vi "Fit VI window to Content__ogtk.vi"(4 "error in (no error)":errorcluster, 6 "border spacing (2 px)":i32=2, 7 "VI Ref (calling VI)":refnum<vi>) -> (0 "error out":errorcluster, 3 "dup VI Ref":refnum<vi>)   [LabVIEW 2017]
doc: "This utility will fit (resize and center) a VI (defined by the \"VI Ref\" input) about the all of the Front Panel object. It will add a border defined by border spacing in units of pixels. If no VI Reference is passed in, it will operate on the calling VI."
uses:
  Close Generic Object Refnum (Array)__ogtk.vi
panel:
  # "Fit VI window to Content.vi\n\nFits a VI's front panel window to its FP Contents.\n\nPlease visit http://www.OpenG.org to learn about the\nOpen Source LabVIEW software movement.\n\nNOTICE -- YOU MUST LEAVE THIS NOTICE IN PLACE.  PER THE TERMS OF THE LICENSE BELOW, YOU MAY SUBLICENSE THIS SOFTWARE \nIN ANY WAY THAT DOES NOT CONFLICT WITH THIS LICENSE.\n\n### BSD License (http://www.opensource.org/licenses/bsd-license.php) Begin ###\n \nCopyright (c) 2002-2004, Jim Kring <jim@jimkring.com>\nCopyright (c) 2002, Cal-Bay Systems, Inc. <info@calbay.com>\n\nAll rights reserved.\n\nRedistribution and use in source and binary forms, with or without modification, are permitted provided that the following conditions are met:\n\n    * Redistributions of source code must retain the above copyright notice, this list of conditions and the following disclaimer.\n    * Redistributions in binary form must reproduce the above copyright notice, this list of conditions and the following disclaimer in the \n       documentation and/or other materials provided with the distribution.\n    * Neither the name of SciWare, James Kring, Inc., nor the names of its contributors may be used to endorse or promote products derived \n       from this software without specific prior written permission.\n\nTHIS SOFTWARE IS PROVIDED BY THE COPYRIGHT HOLDERS AND CONTRIBUTORS \"AS IS\" AND ANY EXPRESS OR IMPLIED WARRANTIES, \nINCLUDING, BUT NOT LIMITED TO, THE IMPLIED WARRANTIES OF MERCHANTABILITY AND FITNESS FOR A PARTICULAR PURPOSE ARE \nDISCLAIMED. IN NO EVENT SHALL THE COPYRIGHT OWNER OR CONTRIBUTORS BE LIABLE FOR ANY DIRECT, INDIRECT, INCIDENTAL,\n SPECIAL, EXEMPLARY, OR CONSEQUENTIAL DAMAGES (INCLUDING, BUT NOT LIMITED TO, PROCUREMENT OF SUBSTITUTE GOODS OR \nSERVICES; LOSS OF USE, DATA, OR PROFITS; OR BUSINESS INTERRUPTION) HOWEVER CAUSED AND ON ANY THEORY OF LIABILITY, \nWHETHER IN CONTRACT, STRICT LIABILITY, OR TORT (INCLUDING NEGLIGENCE OR OTHERWISE) ARISING IN ANY WAY OUT OF THE USE \nOF THIS SOFTWARE, EVEN IF ADVISED OF THE POSSIBILITY OF SUCH DAMAGE.\n\n### BSD License End ###"
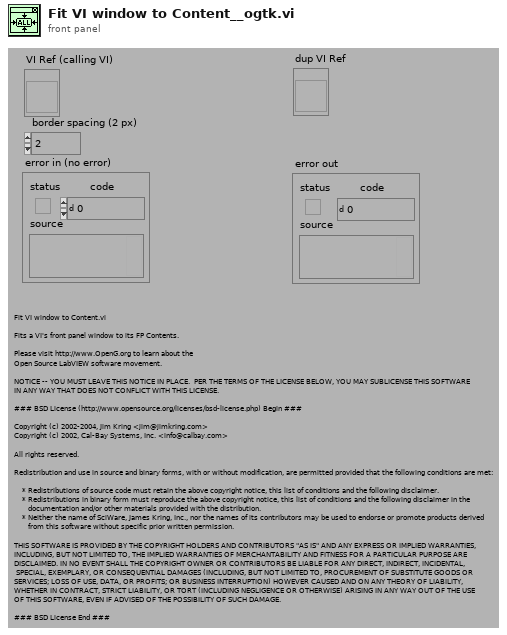
[diagram p1: front panel]
types:
  T1 = typedef "LVRectTypeDef.ctl" = cluster{"Left":i16, "Top":i16, "Right":i16, "Bottom":i16}
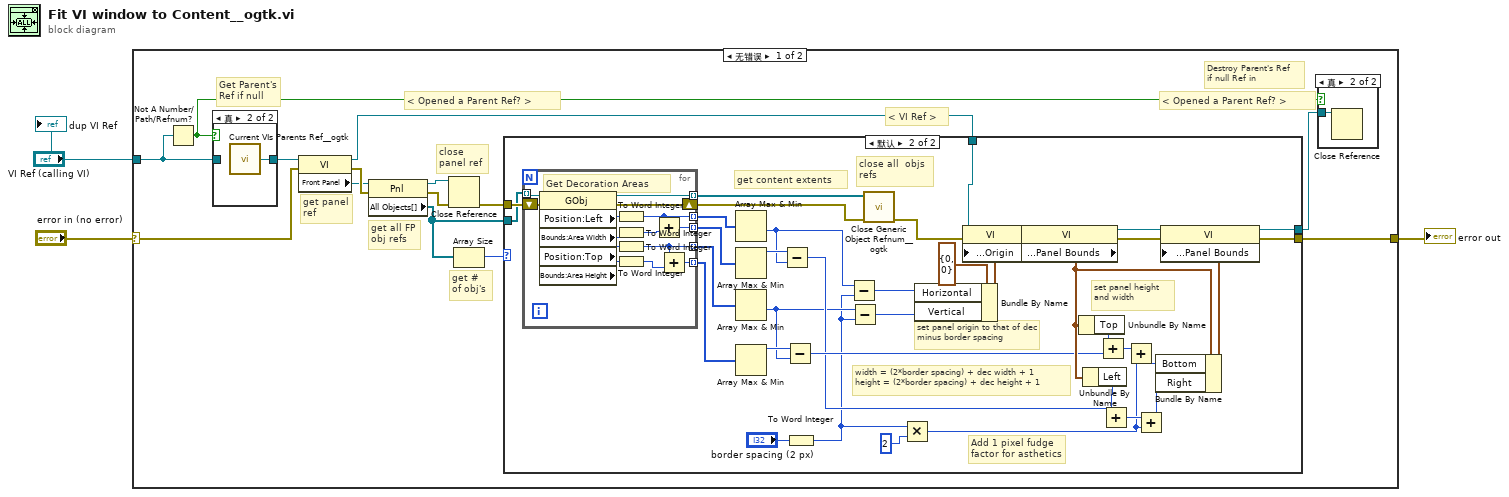
[diagram p0: block diagram]
diagram:
  n1 = case shown="无错误" "error in (no error)" {
    selector: "error in (no error)" -> [w4 w75]
    tunnel: [w11 w75] -> w3
    tunnel: "VI Ref (calling VI)" -> [w5 _]
    frame No Error {
      # "< Opened a Parent Ref? >"
      # "< Opened a Parent Ref? >"
      # "Destroy Parent's Ref\nif null Ref in"
      # "Get Parent's\nRef if null"
      # "get # of obj's"
      # "get panel ref"
      # "get all FP obj refs"
      # "close panel ref"
      # "< VI Ref >"
      n2 = Not A Number/Path/Refnum?(number/path/refnum=w5) -> (NaN/Path/Refnum?=w7:bool)
      n3 = case shown="真" w7 {
        tunnel: [w19 w20] -> w8
        tunnel: w5 -> [w19 _]
        frame False {
        }
        frame True {
          n4 = call "Current VIs Parents Ref__ogtk.vi"() -> ("Calling VI's Reference"=w20:refnum<vi>)  [unwired: 2 in]
        }
      }
      n5 = property on="Property Node" class="VI"(reference=w8, error in=w4) -> (reference out=w17:refnum<vi>, error out=w15:errorcluster, "Front Panel"=w13:refnum<vi>)
      n6 = property on="Property Node" class="Pnl"(reference=w13, error in=w15) -> (reference out=w16:refnum<vi>, error out=w14:errorcluster, "All Objects[]"=w10:refnum<vi>[])
      n7 = Close Reference(reference=w16, error in (no error)=w14) -> (error out=w12:errorcluster)
      n8 = Array Size(array=w10) -> (size(s)=w9:i32)
      n9 = case shown="默认" w9 {
        tunnel: w17 -> [w22 w58]
        tunnel: w12 -> [w21 w45]
        tunnel: [w21 w40] -> w11
        tunnel: [w22 w39] -> w6
        tunnel: w10 -> [_ w38]
        frame 0 {
          # "do nothing if no objects"
        }
        frame Default {
          # "width = (2*border spacing) + dec width + 1\nheight = (2*border spacing) + dec height + 1"
          # "set panel height and width"
          # "set panel origin to that of dec minus border spacing"
          # "close all  objs refs"
          # "get content extents"
          # "Add 1 pixel fudge factor for asthetics"
          n10 = for {
            tunnel: w38 -> [w74] mode=indexing
            shift-right: [w72] -> w25
            shift-left: w45 -> [w73]
            tunnel: [w71] -> w26 mode=indexing
            tunnel: [w67] -> w36 mode=indexing
            tunnel: [w69] -> w35 mode=indexing
            tunnel: [w63] -> w34 mode=indexing
            tunnel: [w68] -> w33 mode=indexing
            # "Get Decoration Areas"
            n11 = property class="GObj"(reference=w74, error in=w73) -> (reference out=w71:refnum<vi>, error out=w72:errorcluster, "Position:Left"=w70:i32, "Bounds:Area Width"=w66:u32, "Position:Top"=w64:i32, "Bounds:Area Height"=w62:u32)
            n12 = To Word Integer(number=w70) -> (16bit integer=w67:i16)
            n13 = To Word Integer(number=w66) -> (16bit integer=w65:i16)
            n14 = To Word Integer(number=w64) -> (16bit integer=w63:i16)
            n15 = To Word Integer(number=w62) -> (16bit integer=w61:i16)
            n16 = Add(x=w67, y=w65) -> (x+y=w69:i16)
            n17 = Add(x=w63, y=w61) -> (x+y=w68:i16)
          }
          n18 = Array Max & Min(array=w36) -> (min value=w27:i16)  [unwired: 3 out]
          n19 = Array Max & Min(array=w35) -> (max value=w30:i16)  [unwired: 3 out]
          n20 = Array Max & Min(array=w34) -> (min value=w28:i16)  [unwired: 3 out]
          n21 = Array Max & Min(array=w33) -> (max value=w32:i16)  [unwired: 3 out]
          n22 = Subtract(x=w30, y=w27) -> (x-y=w29:i16)
          n23 = Subtract(x=w32, y=w28) -> (x-y=w31:i16)
          n24 = To Word Integer(number="border spacing (2 px)") -> (16bit integer=w23:i16)
          n25 = Subtract(x=w27, y=w23) -> (x-y=w48:i16)
          n26 = Subtract(x=w28, y=w23) -> (x-y=w49:i16)
          n27 = call-poly "Close Generic Object Refnum__ogtk.vi"("error in (no error)"=w25, "Gen Refnum Array"=w26) -> ("error out"=w24:errorcluster)  [unwired: 9 in]
          n28 = Multiply(x=w23, y=i16 2) -> (x*y=w37:i16)
          n29 = Bundle By Name(cluster=cluster{"Horizontal":i16, "Vertical":i16} {"Horizontal"=0, "Vertical"=0} ("Front Panel Window:Origin"), "Horizontal"=w48, "Vertical"=w49) -> (w46:cluster{"Horizontal":i16, "Vertical":i16})
          n30 = property on="Property Node" class="VI"(reference=w58, error in=w24, "Front Panel Window:Origin"=w46) -> (reference out=w59:refnum<vi>, error out=w42:errorcluster)
          n31 = property on="Property Node" class="VI"(reference=w59, error in=w42) -> (reference out=w60:refnum<vi>, error out=w41:errorcluster, "Front Panel Window:Panel Bounds"=w50:T1)
          n32 = Unbundle By Name(w50) -> ("Top"=w51:i16)
          n33 = Unbundle By Name(w50) -> ("Left"=w52:i16)
          n34 = Add(x=w51, y=w31) -> (x+y=w56:i16)
          n35 = Add(x=w52, y=w29) -> (x+y=w54:i16)
          n36 = Add(x=w56, y=w37) -> (x+y=w57:i16)
          n37 = Add(x=w54, y=w37) -> (x+y=w55:i16)
          n38 = Bundle By Name(cluster=w50, "Bottom"=w57, "Right"=w55) -> (w53:T1)
          n39 = property on="Property Node" class="VI"(reference=w60, error in=w41, "Front Panel Window:Panel Bounds"=w53) -> (reference out=w39:refnum<vi>, error out=w40:errorcluster)
        }
      }
      n40 = case shown="真" w7 {
        tunnel: w6 -> [_ w18]
        frame False {
        }
        frame True {
          n41 = Close Reference(reference=w18) -> ()  [unwired: 1 in, 1 out]
        }
      }
    }
    frame Error {
    }
  }
  "error out" <- w3
  "dup VI Ref" <- "VI Ref (calling VI)"
